vi "Configure Digitize.vi"(6 "Count (1)":u32=1, 7 "Sample Rate (1E+6)":dbl=1000000.0, 8 "error in (no error)":errorcluster, 9 "Channel List(\"\")":string, 10 "Function (13: Digitize Voltage)":i32(ring)=13 items=["Digitize Voltage"=13, "Digitize Current"=14], 11 "VISA resource name":refnum<visa-resource-name>) -> (0 "error out":errorcluster, 3 "VISA resource name out":refnum<visa-resource-name>)   [LabVIEW 2016, in "Keithley DMM6500 DAQ6500 Series.lvlib"]
doc: "Selects which digitize function is active, sets the number of measurements to digitize when a measurement is requested and defines the precise acquisition rate at which the digitizing measurements are made."
uses:
  Keithley DMM6500 DAQ6500 Series.lvlib
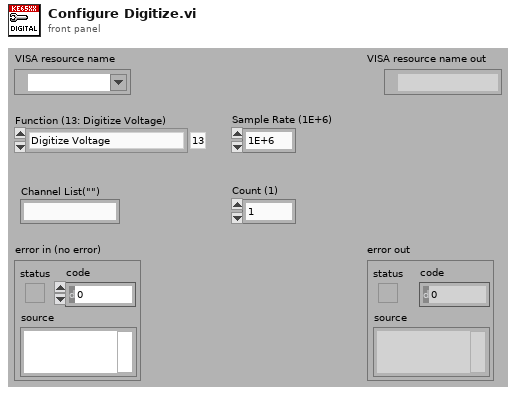
[diagram p1: front panel]
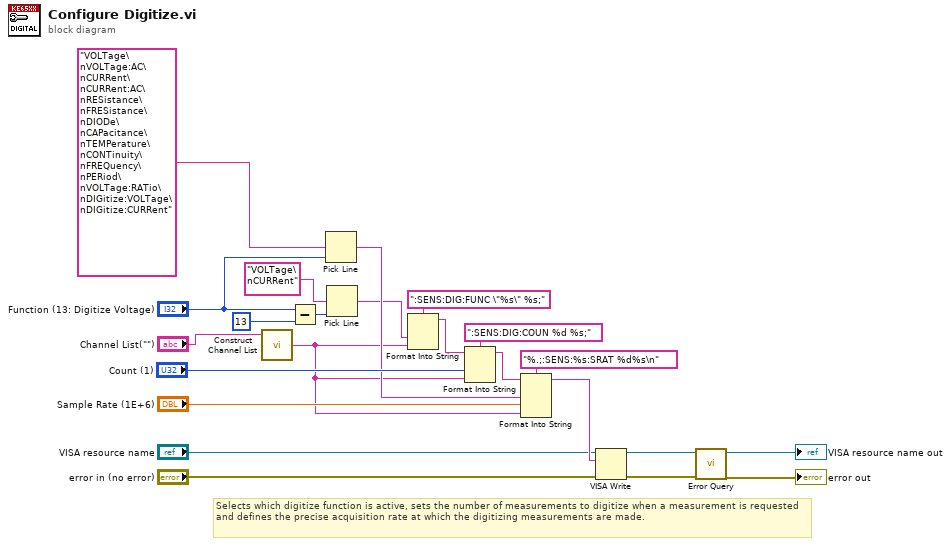
[diagram p0: block diagram]
diagram:
  # "Selects which digitize function is active, sets the number of measurements to digitize when a measurement is requested and defines the precise acquisition rate at which the digitizing measurements are made."
  n1 = call "Construct Channel List.vi"("Channel List"="Channel List(\"\")") -> ("Channel List String"=w1:string)  [unwired: 2 in]
  n2 = Subtract(x="Function (13: Digitize Voltage)", y=13) -> (x-y=w3:i32)
  n3 = Pick Line(multi-line string="VOLTage\nVOLTage:AC\nCURRent\nCURRent:AC\nRESistance\nFRESistance\nDIODe\nCAPacitance\nTEMPerature\nCONTinuity\nFREQuency\nPERiod\nVOLTage:RATio\nDIGitize:VOLTage\nDIGitize:CURRent", line index="Function (13: Digitize Voltage)") -> (output string=w7:string)  [unwired: 1 in]
  n4 = Pick Line(multi-line string="VOLTage\nCURRent", line index=w3) -> (output string=w5:string)  [unwired: 1 in]
  n5 = Format Into String(format string=":SENS:DIG:FUNC \"%s\" %s;", w5, w1) -> (resulting string=w11:string)  [unwired: 2 in, 1 out]
  n6 = Format Into String(format string=":SENS:DIG:COUN %d %s;", initial string=w11, "Count (1)", w1) -> (resulting string=w10:string)  [unwired: 1 in, 1 out]
  n7 = Format Into String(format string="%.;:SENS:%s:SRAT %d%s\n", initial string=w10, w7, "Sample Rate (1E+6)", w1) -> (resulting string=w20:string)  [unwired: 1 in, 1 out]
  n8 = VISA Write(VISA resource name="VISA resource name", write buffer=w20, error in (no error)="error in (no error)") -> (VISA resource name out=w17:refnum<visa-resource-name>, error out=w16:errorcluster)  [unwired: 1 out]
  n9 = call "Error Query.vi"("error in (no error)"=w16, "VISA resource name"=w17) -> ("error out"=→"error out":errorcluster, "VISA resource name out"=→"VISA resource name out":refnum<visa-resource-name>)  [unwired: 6 in, 2 out]
